vi "VFH-data_handle-find_step_change.vi"(10 "data":dbl[](array[numeric])) -> (2 "step points":i32[](array[numeric]))   [LabVIEW 2020, in "VFH-VNA_File_Handler.lvlib"]
uses:
  VFH-VNA_File_Handler.lvlib
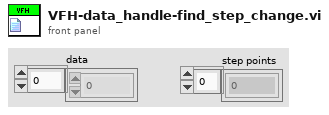
[diagram p1: front panel]
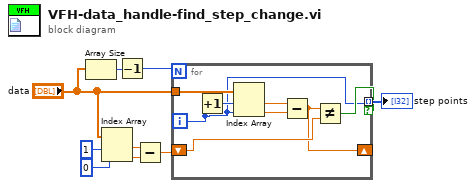
[diagram p0: block diagram]
diagram:
  n1 = Array Size(array="data") -> (size(s)=w9:i32)
  n2 = Index Array(array="data", index #1=1 ("index"), index #2=0 ("index")) -> (element #1=w5:dbl, element #2=w4:dbl)
  n3 = Decrement(x=w9) -> (x-1=w8:i32)
  n4 = Subtract(x=w5, y=w4) -> (x-y=w3:dbl)
  n5 = for {
    N: w8 -> [_]
    tunnel: "data" -> [w17]
    shift-right: [w11] -> _
    shift-left: w3 -> [w13]
    tunnel: [w10] -> w1 mode=indexing if=w12
    i -> [w10]
    n6 = Increment(x=w10) -> (x+1=w14:i32)
    n7 = Index Array(array=w17, index #1=w14, index #2=w10) -> (element #1=w15:dbl, element #2=w16:dbl)
    n8 = Subtract(x=w15, y=w16) -> (x-y=w11:dbl)
    n9 = Not Equal?(x=w11, y=w13) -> (x != y?=w12:bool)
  }
  "step points" <- w1
